vi "Read.vi"(8 "error in (no error)":errorcluster caption="entrée d'erreur (pas d'erreur)", 11 "Server TCP_IP (Default) en entrée":refnum<class "Client TCP_IP (Default).lvclass">) -> (0 "error out":errorcluster caption="sortie d'erreur", 3 "Server TCP_IP (Default) en sortie":refnum<class "Client TCP_IP (Default).lvclass">)   [LabVIEW 2020, in "Library Instrument & Equipement.lvlib" / "Library TCP IP.lvlib" / "Client TCP_IP (Default).lvclass"]
uses:
  Client TCP_IP (Default).lvclass
  Client TCP_IP (Default).lvclass/Client TCP_IP (Default).ctl
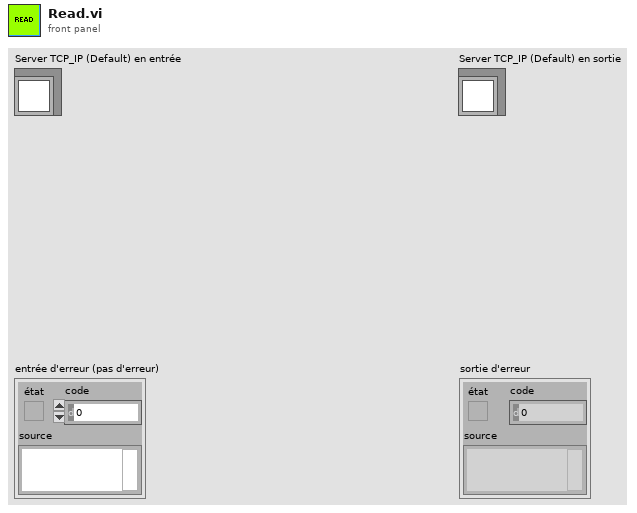
[diagram p1: front panel]
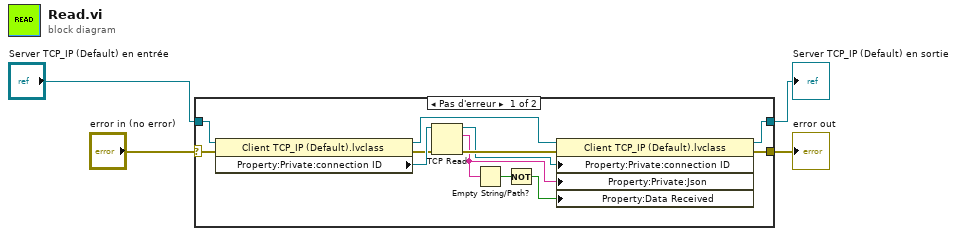
[diagram p0: block diagram]
diagram:
  n1 = case shown="Pas d'erreur" "error in (no error)" {
    selector: "error in (no error)" -> [w10 w18]
    tunnel: [w9 w18] -> w3
    tunnel: [w11 w17] -> w1
    tunnel: "Server TCP_IP (Default) en entrée" -> [w12 w17]
    frame No Error {
      n2 = property class="Client TCP_IP (Default).lvclass"(reference=w12, error in=w10) -> (reference out=w13:refnum<class "Client TCP_IP (Default).lvclass">, error out=w15:errorcluster, "Property:Private:connection ID"=w16:refnum<k5>)
      n3 = TCP Read(connection ID=w16, error in (no error)=w15) -> (connection ID out=w5:refnum<k5>, data out=w8:string, error out=w14:errorcluster)  [unwired: 3 in]
      n4 = Empty String/Path?(string/path=w8) -> (empty?=w7:bool)
      n5 = Not(x=w7) -> (.not. x?=w6:bool)
      n6 = property class="Client TCP_IP (Default).lvclass"(reference=w13, error in=w14, "Property:Private:connection ID"=w5, "Property:Private:Json"=w8, "Property:Data Received"=w6) -> (reference out=w11:refnum<class "Client TCP_IP (Default).lvclass">, error out=w9:errorcluster)
    }
    frame Error {
    }
  }
  "error out" <- w3
  "Server TCP_IP (Default) en sortie" <- w1
